vi "Load Framework.vi"(8 "error in (no error)":errorcluster, 11 "Application Refs":T1={"Item Tree Control"=refnum, "Top-Level VI"=refnum, "menu reference"=refnum, "queue"=refnum, "Stop Pointer"=refnum, "Buffer Variant"=variant, "server ID"=refnum, "framework tag"="", "Values"=refnum, "Hex"=refnum, "ASCII"=refnum, "lines visible"=0, "values padding"=0, "current buffer data"={"decimation"=0, "avg bandwidth"=0.0, "channels"=[], "byte order"=enum."little-endian", "buffer descriptor"={"buffer type"=enum."Engine", "plugin id"=0, "group id"=0, "transfer id"=0, "offset"=0, "length"=0}, "values channels"={"index"=0, "count"=0, "engine offset"=0}, "select start offset"=18446744073709551615, "select end offset"=0, "channel index"=-1}, "Framework Configuration"=refnum} {"current buffer data"."channels"."configuration"."string offset" format="%d bytes"; "current buffer data"."avg bandwidth" format="%.0g bytes"}) -> (0 "error out":errorcluster, 3 "Application Data out":T1={"Item Tree Control"=refnum, "Top-Level VI"=refnum, "menu reference"=refnum, "queue"=refnum, "Stop Pointer"=refnum, "Buffer Variant"=variant, "server ID"=refnum, "framework tag"="", "Values"=refnum, "Hex"=refnum, "ASCII"=refnum, "lines visible"=0, "values padding"=0, "current buffer data"={"decimation"=0, "avg bandwidth"=0.0, "channels"=[], "byte order"=enum."little-endian", "buffer descriptor"={"buffer type"=enum."Engine", "plugin id"=0, "group id"=0, "transfer id"=0, "offset"=0, "length"=0}, "values channels"={"index"=0, "count"=0, "engine offset"=0}, "select start offset"=18446744073709551615, "select end offset"=0, "channel index"=-1}, "Framework Configuration"=refnum} {"current buffer data"."channels"."configuration"."string offset" format="%d bytes"; "current buffer data"."avg bandwidth" format="%.0g bytes"})   [LabVIEW 2020, in "DSF Core.lvlib"]
uses:
  DSF Core.lvlib
  Application Data.ctl
  Buffer Reader/Buffer Data.ctl
  <vilib>/NI/Memory Manager/Classes/Pointer/Pointer.lvclass
  Typedefs/DSF Settings Info.ctl
  Typedefs/DSF Byte Order.ctl
  Typedefs/DSF Data Type.ctl
  Typedefs/DSF Buffer Type.ctl
  Classes/Thread/Data Server/DSF Buffer Subset Descriptor.ctl
  Buffer Reader/Queue Data.ctl
  Values Channels.ctl
  Typedefs/Core Channel Configuration.ctl
  Classes/Configuration/Core/Channel/Channel Configuration.lvclass
  Classes/Configuration/Core/Framework/Framework Configuration.lvclass
  Classes/Configuration/Core/Transfer/Channel Configuration.ctl
  Classes/Configuration/Core/Transfer/Transfer Configuration.lvclass
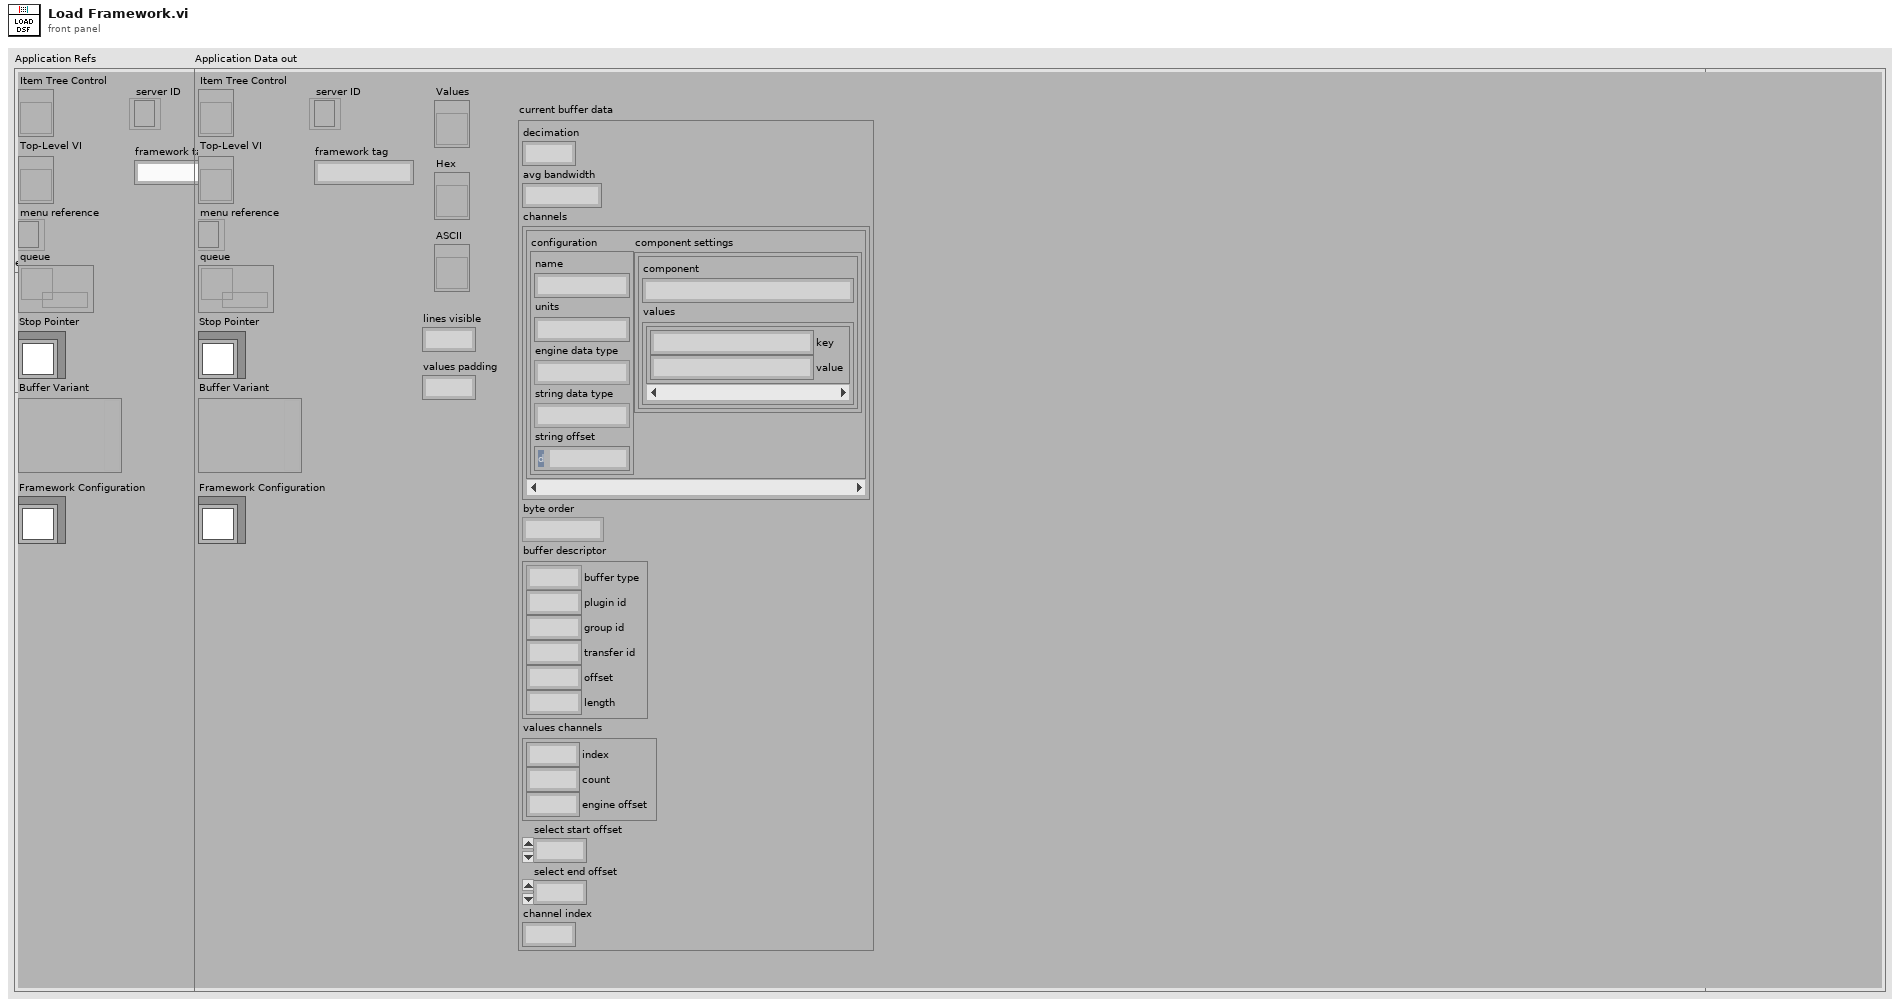
[diagram p1: front panel]
types:
  T1 = typedef "DSF Core.lvlib/Application Data.ctl" = cluster{"Item Tree Control":refnum<vi>, "Top-Level VI":refnum<vi>, "menu reference":refnum<k9>, "queue":refnum<queue>, "Stop Pointer":refnum<class "Pointer.lvclass">, "Buffer Variant":variant, "server ID":refnum<k5>, "framework tag":string, "Values":refnum<vi>, "Hex":refnum<vi>, "ASCII":refnum<vi>, "lines visible":i32, "values padding":i32, "current buffer data":T2, "Framework Configuration":refnum<class "Framework Configuration.lvclass">}
  T2 = typedef "DSF Core.lvlib/Buffer Data.ctl" = cluster{"decimation":u64, "avg bandwidth":dbl, "channels":T3[], "byte order":T7, "buffer descriptor":T8, "values channels":T10, "select start offset":u64, "select end offset":u64, "channel index":i32}
  T3 = typedef "DSF Core.lvlib/Transfer Configuration.lvclass/Channel Configuration.ctl" = cluster{"configuration":T4, "component settings":T6[]}
  T4 = typedef "DSF Core.lvlib/Channel Configuration.lvclass/Core Channel Configuration.ctl" = cluster{"name":string, "units":string, "engine data type":T5, "string data type":T5, "string offset":u64}
  T5 = typedef "DSF Core.lvlib/DSF Data Type.ctl" = enum8{"Bool", "SGL", "DBL", "I8", "I16", "I32", "I64", "U8", "U16", "U32", "U64"}
  T6 = typedef "DSF Core.lvlib/DSF Settings Info.ctl" = cluster{"component":string, "values":cluster{"key":string, "value":string}[]}
  T7 = typedef "DSF Core.lvlib/DSF Byte Order.ctl" = enum8{"big-endian", "little-endian"}
  T8 = typedef "DSF Core.lvlib/DSF Buffer Subset Descriptor.ctl" = cluster{"buffer type":T9, "plugin id":i32, "group id":i32, "transfer id":i32, "offset":u64, "length":i64}
  T9 = typedef "DSF Core.lvlib/DSF Buffer Type.ctl" = enum16{"Engine", "String"}
  T10 = typedef "DSF Core.lvlib/Values Channels.ctl" = cluster{"index":i32, "count":i32, "engine offset":u64}
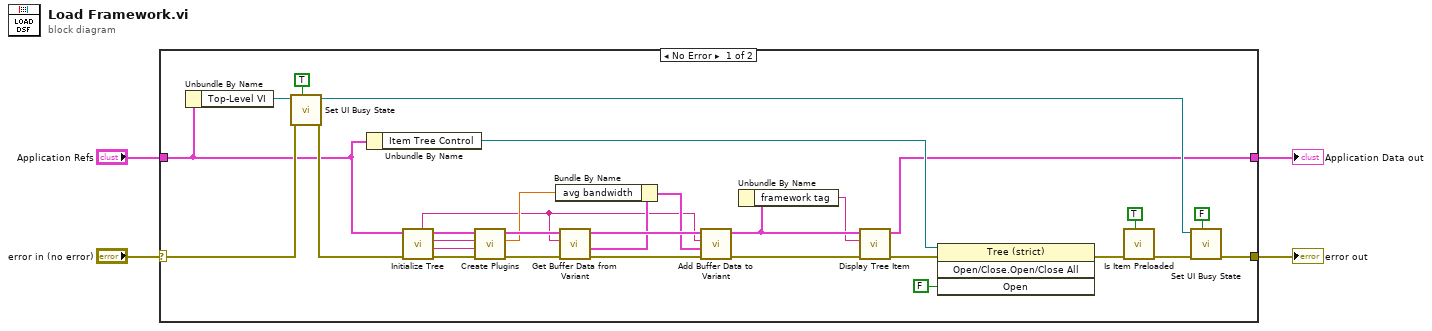
[diagram p0: block diagram]
diagram:
  n1 = case shown="No Error" "error in (no error)" {
    selector: "error in (no error)" -> [w13 w36]
    tunnel: [w7 w35] -> w4
    tunnel: [w14 w36] -> w3
    tunnel: "Application Refs" -> [w10 w35]
    frame No Error {
      n2 = Unbundle By Name(w10) -> ("Top-Level VI"=w19:refnum<vi>)
      n3 = call "Set UI Busy State.vi"("Defer Panel Updates"=TRUE, "error in (no error)"=w13, "VI in"=w19) -> ("error out"=w17:errorcluster, "VI out"=w12:refnum<vi>)  [unwired: 7 in]
      n4 = Unbundle By Name(w10) -> ("Item Tree Control"=w11:refnum<vi>)
      n5 = call "Initialize Tree.vi"("error in (no error)"=w17, "Application Data in"=w10) -> ("error out"=w32:errorcluster, "async plugins tag"=w30:string, "inline plugins tag"=w31:string, "Application Data out"=w33:T1, "framework tag"=w20:string)  [unwired: 5 in]
      n6 = call "Create Plugins.vi"("error in (no error)"=w32, "async plugins tag"=w30, "inline plugins tag"=w31, "Application Data In"=w33) -> ("error out"=w27:errorcluster, "avg bandwidth"=w22:dbl, "Application Data out"=w26:T1)  [unwired: 5 in]
      n7 = call "Get Buffer Data from Variant.vi"("error in (no error)"=w27, "tag"=w20, "Application Data In in"=w26) -> ("error out"=w24:errorcluster, "Buffer data"=w23:T2, "Application Data In out"=w25:T1)  [unwired: 6 in]
      n8 = Bundle By Name(cluster=w23, "avg bandwidth"=w22) -> (w21:T2)
      n9 = call "Add Buffer Data to Variant.vi"("error in (no error)"=w24, "Buffer data"=w21, "tag"=w20, "Application Data In in"=w25) -> ("error out"=w9:errorcluster, "Application Data In out"=w8:T1)  [unwired: 6 in]
      n10 = Unbundle By Name(w8) -> ("framework tag"=w5:string)
      n11 = call "Display Tree Item.vi"("error in (no error)"=w9, "Tag"=w5, "Application Data in"=w8) -> ("error out"=w6:errorcluster, "Application Data out"=w7:T1)  [unwired: 7 in]
      n12 = invoke class="Tree (strict)" method="Open/Close.Open/Close All"(reference=w11, error in=w6, "Open"=FALSE ("Open?")) -> (error out=w28:errorcluster)  [unwired: 1 in, 3 out]
      n13 = call "Is Item Preloaded.vi"("clear entries"=TRUE, "error in (no error)"=w28) -> ("error out"=w15:errorcluster)  [unwired: 7 in, 2 out]
      n14 = call "Set UI Busy State.vi"("Defer Panel Updates"=FALSE, "error in (no error)"=w15, "VI in"=w12) -> ("error out"=w14:errorcluster)  [unwired: 7 in, 1 out]
    }
    frame Error {
    }
  }
  "error out" <- w3
  "Application Data out" <- w4
